vi "State_Machine.vi"(8 "error in (no error)":errorcluster caption="entrée d'erreur (pas d'erreur)", 11 "Flash_Jlink en entrée":refnum<class "Flash_Jlink.lvclass">) -> (0 "error out":errorcluster caption="sortie d'erreur", 2 "Json_String":string, 3 "Flash_Jlink en sortie":refnum<class "Flash_Jlink.lvclass">)   [LabVIEW 2020, in "Library Test.lvlib" / "Flash_Jlink.lvclass"]
uses:
  Flash_Jlink.lvclass
  C:/Users/ngarcin/OneDrive - Altyor/Standard TB/Class/Test/Test (Default)/Test (Default).lvclass
  Flash_Jlink.lvclass/Flash_Jlink.ctl
  Process/Process (Default)/Process (Default).lvclass
panel:
  out "String In progress":string
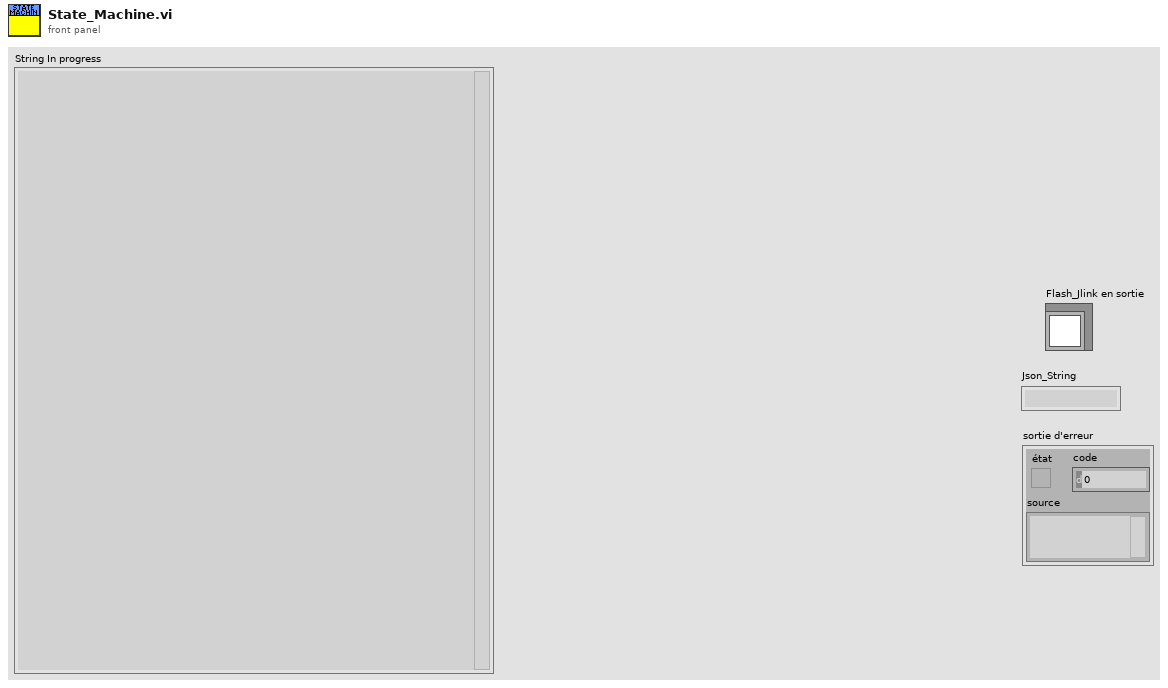
[diagram p1: front panel]
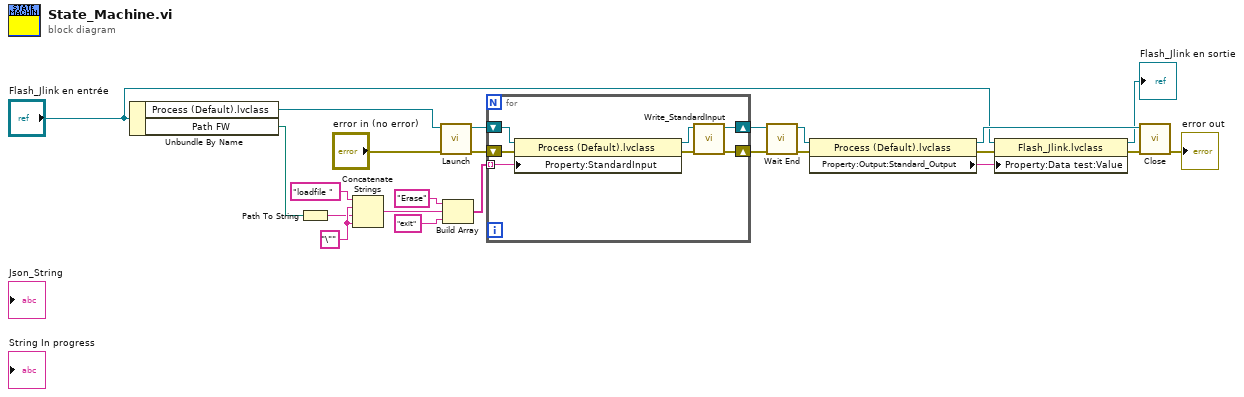
[diagram p0: block diagram]
diagram:
  w18 = "\"" ("chaîne")
  n1 = Unbundle By Name("Flash_Jlink en entrée") -> ("Process (Default).lvclass"=w23:refnum<class "Process (Default).lvclass">, "Path FW"=w9:path)
  n2 = Path To String(path=w9) -> (string=w8:string)
  n3 = Concatenate Strings("loadfile " ("chaîne"), w18, w8, w18) -> (w17:string)
  n4 = call-dynamic "Launch.vi"("error in (no error)"="error in (no error)", "Process (Default) en entrée"=w23) -> ("error out"=w14:errorcluster, "Process (Default) en sortie"=w15:refnum<class "Process (Default).lvclass">)  [unwired: 8 in]
  n5 = Build Array("Erase" ("élément"), w17, "exit" ("élément")) -> (w13:string[])
  n6 = for {
    shift-right: [w30] -> w22
    shift-left: w15 -> [w28]
    shift-right: [w29] -> w21
    shift-left: w14 -> [w26]
    tunnel: w13 -> [w24] mode=indexing
    n7 = property class="Process (Default).lvclass"(reference=w28, error in=w26, "Property:StandardInput"=w24) -> (reference out=w27:refnum<class "Process (Default).lvclass">, error out=w25:errorcluster)
    n8 = call-dynamic "Write_StandardInput.vi"("error in (no error)"=w25, "Process (Default) en entrée"=w27) -> ("error out"=w29:errorcluster, "Process (Default) en sortie"=w30:refnum<class "Process (Default).lvclass">)  [unwired: 8 in]
  }
  n9 = call-dynamic "Wait End.vi"("error in (no error)"=w21, "Process (Default) en entrée"=w22) -> ("error out"=w3:errorcluster, "Process (Default) en sortie"=w12:refnum<class "Process (Default).lvclass">)  [unwired: 8 in]
  n10 = property class="Process (Default).lvclass"(reference=w12, error in=w3) -> (reference out=w11:refnum<class "Process (Default).lvclass">, error out=w5:errorcluster, "Property:Output:Standard_Output"=w4:string)
  n11 = property class="Flash_Jlink.lvclass"(reference="Flash_Jlink en entrée", error in=w5, "Property:Data test:Value"=w4) -> (reference out=→"Flash_Jlink en sortie":refnum<class "Flash_Jlink.lvclass">, error out=w2:errorcluster)
  n12 = call-dynamic "Close.vi"("error in (no error)"=w2, "Process (Default) en entrée"=w11) -> ("error out"=→"error out":errorcluster)  [unwired: 8 in, 1 out]
